vi "Use Software Adjust on Measurements.vi"() -> ()   [LabVIEW 2018]
doc: "Paul Packebush"
uses:
  Global.gbl
  AI Read (scaled array).vi
  <vilib>/Analysis/NI_AALBase.lvlib
  <vilib>/Analysis/baseanly.llb/Mean (DBL).vi
panel:
  out "mean":dbl format="%.5f"
  out "Adjusted Data":dbl(graph)=25.003978177037776
  in  "number of scans to acquire (1000)":i32=100
  in  "scan rate\n(4000 scans/sec)":sgl=1000.0 format="%.2f"
  in  "channels (0)":string[](array[string])=["temp"]
  in  "device (1)":i16=1
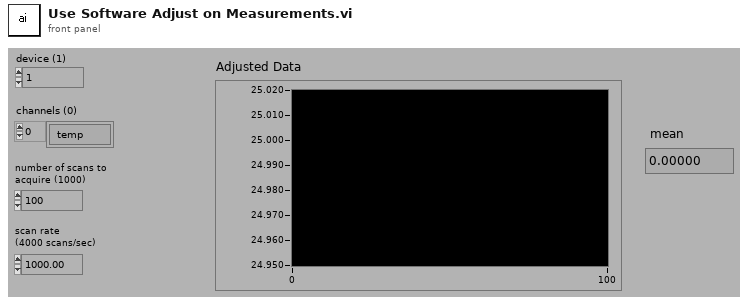
[diagram p1: front panel]
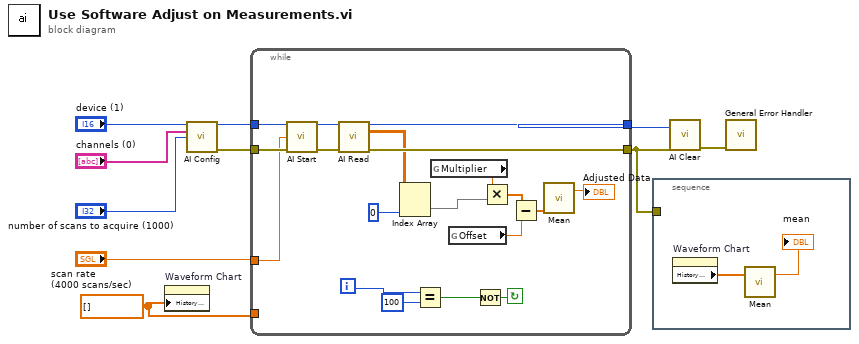
[diagram p0: block diagram]
diagram:
  w1 = dbl[] [] ("Write Attribute")
  n1 = property on="Waveform Chart" class="WFChart (strict)"("History Data"=w1) -> ()  [unwired: 2 in, 2 out]
  n2 = call "AI Config.vi"("device (1)"="device (1)", "channels (0)"="channels (0)", "buffer size (1000 scans)"="number of scans to acquire (1000)") -> ("taskID"=w6:u32, "error out"=w10:errorcluster)  [unwired: 10 in, 1 out]
  n3 = while {
    tunnel: w1 -> [_]
    tunnel: "scan rate\n(4000 scans/sec)" -> [w20]
    tunnel: [w24] -> w3
    tunnel: w6 -> [w26]
    tunnel: [w27] -> w9
    tunnel: w10 -> [w28]
    i -> [w19]
    stop <- w11 continue-if-true
    n4 = call "AI Start.vi"("taskID in"=w26, "scan rate (1000 scans/sec)"=w20, "error in (no error)"=w28) -> ("taskID out"=w25:u32, "error out"=w29:errorcluster)  [unwired: 9 in, 2 out]
    n5 = call-poly "AI Read.vi"("taskID in"=w25, "error in (no error)"=w29) -> ("taskID out"=w27:u32, "scaled data"=w23:sgl[][], "error out"=w24:errorcluster)  [unwired: 8 in, 3 out]
    n6 = Index Array(array=w23, index (col)=0 ("Index")) -> (element=w17:sgl[])  [unwired: 1 in]
    n7 = Equal?(x=w19, y=100) -> (x = y?=w12:bool)
    n8 = global read "Global.gbl" "Multiplier"() -> (w13:dbl)
    n9 = global read "Global.gbl" "Offset"() -> (w15:dbl)
    n10 = Not(x=w12) -> (.not. x?=w11:bool)
    n11 = Multiply(x=w13, y=w17) -> (x*y=w16:dbl[])
    n12 = Subtract(x=w16, y=w15) -> (x-y=w14:dbl[])
    n13 = call-poly <vilib>:"Mean.vi"("X"=w14) -> ("mean"=→"Adjusted Data":dbl)  [unwired: 1 out]
  }
  n14 = stacked-sequence {
    tunnel: w3 -> [_]
    frame #0 {
      n15 = property on="Waveform Chart" class="WFChart (strict)"() -> ("History Data"=w31:dbl[])  [unwired: 2 in, 2 out]
      n16 = call-poly <vilib>:"Mean.vi"("X"=w31) -> ("mean"=→"mean":dbl)  [unwired: 1 out]
    }
  }
  n17 = call "AI Clear.vi"("error in (no error)"=w3, "taskID in"=w9) -> ("error out"=w5:errorcluster)  [unwired: 4 in, 1 out]
  n18 = call <vilib>:"General Error Handler.vi"("error in (no error)"=w5) -> ()  [unwired: 10 in, 5 out]
